vi "ALTS-2015 OPC Engine Globals.vi"() -> ()   [LabVIEW 2013]
panel:
  in  "OPC Exit?":bool
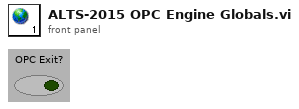
[diagram p1: front panel]
diagram:
